vi "Targeting VI.vi"(0 "Upper Limit":T1, 4 "Lower Limit":T1, 6 "RobotDriveDevRef":T7={"DevStatus"={"status"=FALSE, "code"=0, "source"=""}, "Motors[]"=[], "Square Inputs"=FALSE, "Max Output"=1.0, "Isochronous"=FALSE}, 7 "Elevator Control":T8={"DeviceStatus"={"status"=FALSE, "code"=0, "source"=""}, "Type"=enum."PWM", "PWM"={"Digital Module"=enum."Digital Module 1", "PWM Channel"=enum."Invalid", "DeadBand"={"Name"="", "maxPositivePwm"=0, "minPositivePwm"=0, "centerPwm"=0, "maxNegativePwm"=0, "minNegativePwm"=0, "angularRange"=0}}, "CAN"={"Device Number"=0, "Control Mode"=enum."Percent VBus", "Semaphore"=refnum, "Max Vout"=12.0}, "Invert"=FALSE, "TransformRef"=refnum, "InvTransformRef"=refnum}, 8 "DO 14 LED":T14, 9 "Shoot":T4={"DevStatus"={"status"=FALSE, "code"=0, "source"=""}, "Solenoid Module"=enum."Solenoid Module 1", "Forward Solenoid Channel"=enum."Invalid", "Reverse Solenoid Channel"=enum."Invalid"}, 10 "slow turn":dbl=0.5, 11 "Aim Button":bool) -> ()   [LabVIEW 2012]
uses:
  <vilib>/Rock Robotics/WPI/DigitalOutput/WPI_DigitalOutputDevRef.ctl
  <vilib>/Rock Robotics/SystemInterfaces/Typedef/FPGA_TypedefDigitalModule.ctl
  <vilib>/Rock Robotics/SystemInterfaces/DIO/FPGA_DIOChannel.ctl
  <vilib>/Rock Robotics/WPI/MotorControl/WPI_MotorControlDeviceRef.ctl
  <vilib>/Rock Robotics/SystemInterfaces/DIO/FPGA_DIOPWMChannel.ctl
  <vilib>/Rock Robotics/WPI/PWM/WPI_PWMDeadband.ctl
  <vilib>/Rock Robotics/WPI/CAN/Jaguar/SubVIs/WPI_CANJaguar_ControlMode.ctl
  <vilib>/Rock Robotics/WPI/PWM/WPI_PWMTransform_ConPane.ctl
  <vilib>/Rock Robotics/WPI/RobotDrive/WPI_RobotDriveDevRef.ctl
  <vilib>/Rock Robotics/WPI/Solenoid/WPI_SolenoidDevRef.ctl
  <vilib>/Rock Robotics/SystemInterfaces/Typedef/FPGA_TypedefSolenoidModule.ctl
  <vilib>/Rock Robotics/WPI/Solenoid/WPI_SolenoidChannel.ctl
  <vilib>/Rock Robotics/WPI/DigitalInput/WPI_DigitalInputDevRef.ctl
  <vilib>/Rock Robotics/WPI/Solenoid/WPI_SolenoidValue.ctl
  Robot Global Data.vi
  <vilib>/Rock Robotics/WPI/Solenoid/WPI_SolenoidSetEnum.vi
panel:
  in  "lower limit Y":dbl=0.48
  in  "upper limit Y":dbl=0.5
  in  "upper limit X":dbl=0.1
  in  "lower limit X":dbl=-0.1
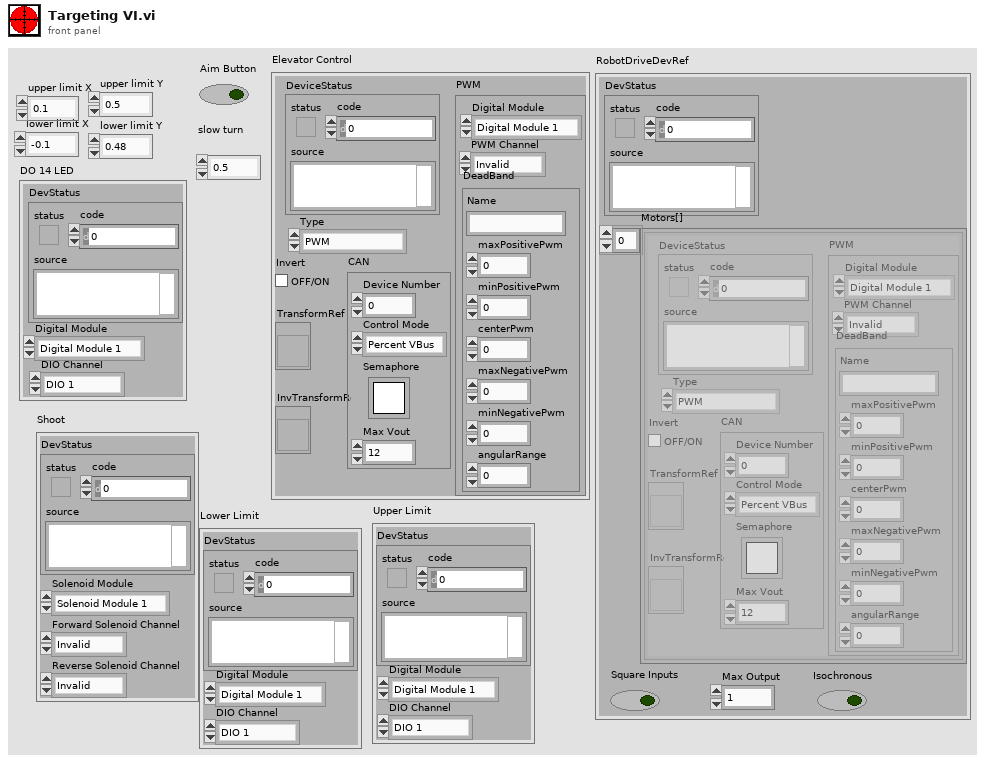
[diagram p1: front panel]
types:
  T1 = typedef "WPI_DigitalInputDevRef.ctl" = cluster{"DevStatus":errorcluster, "DIO Channel":T2, "Digital Module":T3}
  T2 = typedef "FPGA_DIOChannel.ctl" = enum8{"DIO 1", "DIO 2", "DIO 3", "DIO 4", "DIO 5", "DIO 6", "DIO 7", "DIO 8", "DIO 9", "DIO 10", "DIO 11", "DIO 12", "DIO 13", "DIO 14", "Invalid"}
  T3 = typedef "FPGA_TypedefDigitalModule.ctl" = enum16{"Digital Module 1", "Digital Module 2"}
  T4 = typedef "WPI_SolenoidDevRef.ctl" = cluster{"DevStatus":errorcluster, "Solenoid Module":T5, "Forward Solenoid Channel":T6, "Reverse Solenoid Channel":T6}
  T5 = typedef "FPGA_TypedefSolenoidModule.ctl" = enum16{"Solenoid Module 1", "Solenoid Module 2"}
  T6 = typedef "WPI_SolenoidChannel.ctl" = enum8{"Solenoid 1", "Solenoid 2", "Solenoid 3", "Solenoid 4", "Solenoid 5", "Solenoid 6", "Solenoid 7", "Solenoid 8", "Invalid"}
  T7 = typedef "WPI_RobotDriveDevRef.ctl" = cluster{"DevStatus":errorcluster, "Motors[]":T8[], "Square Inputs":bool, "Max Output":dbl, "Isochronous":bool}
  T8 = typedef "WPI_MotorControlDeviceRef.ctl" = cluster{"DeviceStatus":errorcluster, "Type":enum16{"PWM", "CAN"}, "PWM":cluster{"Digital Module":T3, "PWM Channel":T9, "DeadBand":T10}, "CAN":cluster{"Device Number":u8, "Control Mode":T11, "Semaphore":T12, "Max Vout":dbl}, "Invert":bool, "TransformRef":T13, "InvTransformRef":T13}
  T9 = typedef "FPGA_DIOPWMChannel.ctl" = enum8{"PWM 1", "PWM 2", "PWM 3", "PWM 4", "PWM 5", "PWM 6", "PWM 7", "PWM 8", "PWM 9", "PWM 10", "Invalid"}
  T10 = typedef "WPI_PWMDeadband.ctl" = cluster{"Name":string, "maxPositivePwm":i32, "minPositivePwm":i32, "centerPwm":i32, "maxNegativePwm":i32, "minNegativePwm":i32, "angularRange":u16}
  T11 = typedef "WPI_CANJaguar_ControlMode.ctl" = enum8{"Percent VBus", "Current", "Speed", "Position", "Voltage"}
  T12 = typedef "Semaphore RefNum" = refnum<k1>
  T13 = typedef "WPI_PWMTransform_ConPane.ctl" = refnum<vi>
  T14 = typedef "WPI_DigitalOutputDevRef.ctl" = cluster{"Digital Module":T3, "DIO Channel":T2, "DevStatus":errorcluster}
  T15 = cluster{"Center Position":cluster{"X":dbl, "Y":dbl}, "Distance (ft)":dbl, "Center":bool}[]
  T16 = cluster{"Center Position":cluster{"X":dbl, "Y":dbl}, "Distance (ft)":dbl, "Center":bool}
  T17 = typedef "WPI_SolenoidValue.ctl" = enum16{"Off", "On", "Forward", "Reverse"}
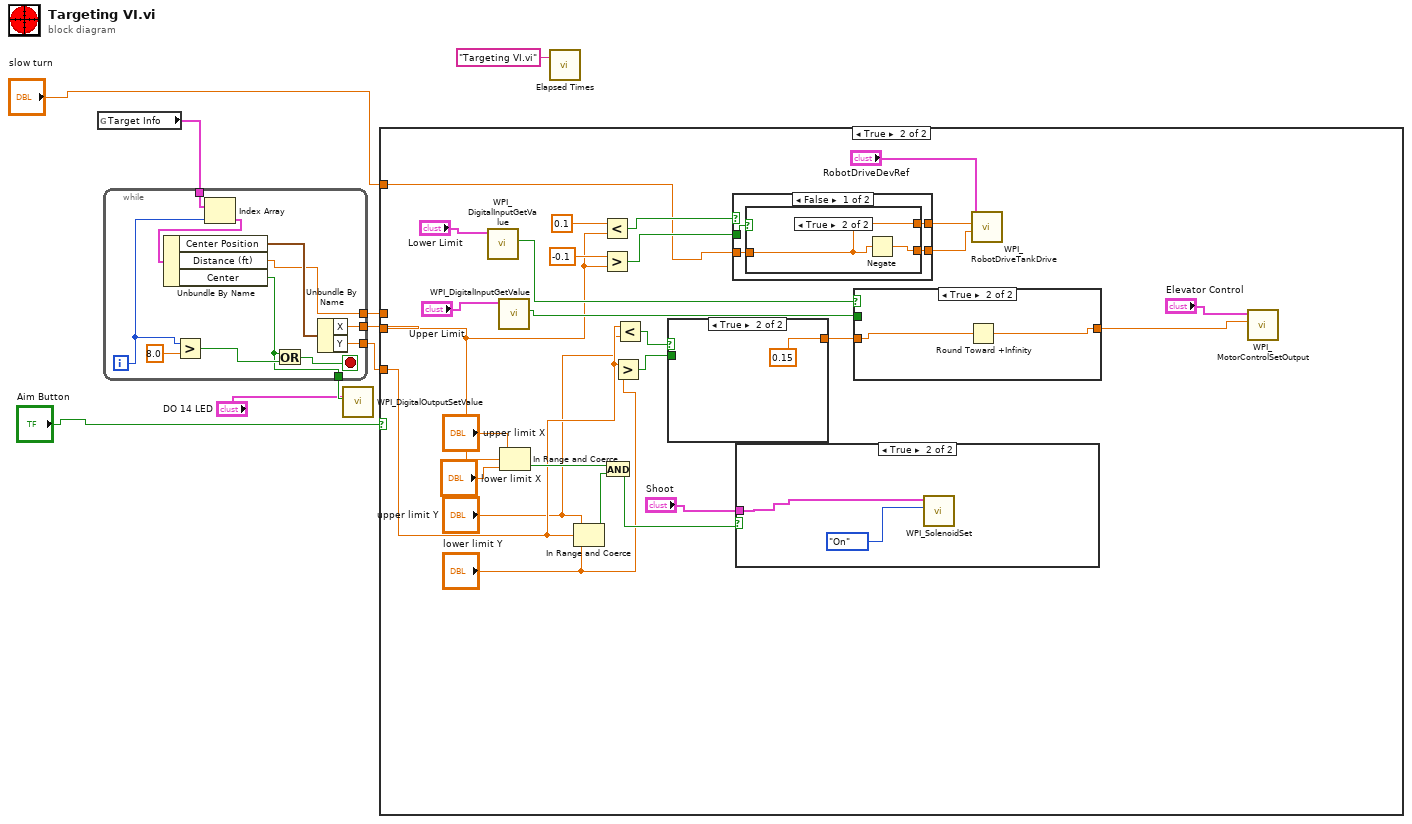
[diagram p0: block diagram]
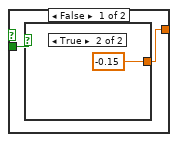
[diagram p3: hidden frame]
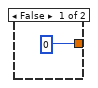
[diagram p4: hidden frame]
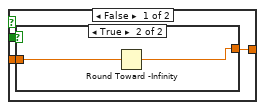
[diagram p5: hidden frame]
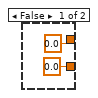
[diagram p7: hidden frame]
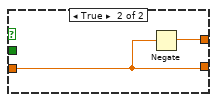
[diagram p8: hidden frame]
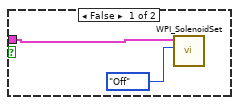
[diagram p9: hidden frame]
diagram:
  n1 = global read "Robot Global Data.vi" "Target Info"() -> (w9:T15)
  n2 = while {
    tunnel: [w19] -> w7
    tunnel: [w18] -> w6
    tunnel: w9 -> [w17]
    tunnel: [w11] -> w8
    tunnel: [w10] -> w1
    i -> [w12]
    stop <- w15 stop-if-true
    n3 = Greater?(x=w12, y=8.0) -> (0:w14:bool)
    n4 = Index Array(array=w17, index=w12) -> (element=w16:T16)
    n5 = Unbundle By Name(w16) -> ("Center Position"=w20:cluster{"X":dbl, "Y":dbl}, "Distance (ft)"=w10:dbl, "Center"=w11:bool)
    n6 = Or(x=w11, y=w14) -> (x .or. y?=w15:bool)
    n7 = Unbundle By Name(w20) -> ("X"=w18:dbl, "Y"=w19:dbl)
  }
  n8 = call <vilib>:"WPI_DigitalOutputSetValue.vi"("Value"=w8, "DigitalOutputDevRef"="DO 14 LED") -> ()  [unwired: 8 in, 2 out]
  n9 = case shown="True" "Aim Button" {
    tunnel: w7 -> [_ w23]
    tunnel: w6 -> [_ w37]
    tunnel: "slow turn" -> [_ w40]
    tunnel: w1 -> [_ _]
    frame False {
    }
    frame True {
      n10 = call <vilib>:"WPI_DigitalInputGetValue.vi"("DigitalInputDevRef"="Lower Limit") -> ("Value"=w39:bool)  [unwired: 8 in, 2 out]
      n11 = call <vilib>:"WPI_DigitalInputGetValue.vi"("DigitalInputDevRef"="Upper Limit") -> ("Value"=w38:bool)  [unwired: 8 in, 2 out]
      n12 = In Range and Coerce(upper limit="upper limit X", x=w37, lower limit="lower limit X") -> (In Range?=w35:bool)  [unwired: 1 out]
      n13 = In Range and Coerce(upper limit="upper limit Y", x=w23, lower limit="lower limit Y") -> (In Range?=w36:bool)  [unwired: 1 out]
      n14 = Less?(x=0.1, y=w37) -> (x < y?=w42:bool)
      n15 = Greater?(x=-0.1, y=w37) -> (0:w41:bool)
      n16 = And(x=w35, y=w36) -> (x .and. y?=w43:bool)
      n17 = Greater?(x=w23, y="lower limit Y") -> (0:w25:bool)
      n18 = Less?(x=w23, y="upper limit Y") -> (x < y?=w26:bool)
      n19 = case shown="True" w26 {
        tunnel: w25 -> [w49 _]
        tunnel: [w48 0.15] -> w24
        frame False {
          n20 = case shown="True" w49 {
            tunnel: [0 -0.15] -> w48
            frame False {
            }
            frame True {
            }
          }
        }
        frame True {
        }
      }
      n21 = case shown="False" w42 {
        tunnel: [w64 w70] -> w45
        tunnel: [w62 w69] -> w44
        tunnel: w40 -> [w63 w69]
        tunnel: w41 -> [w61 _]
        frame False {
          n22 = case shown="True" w61 {
            tunnel: [0.0 w67] -> w64
            tunnel: w63 -> [_ w67]
            tunnel: [0.0 w68] -> w62
            frame False {
            }
            frame True {
              n23 = Negate(x=w67) -> (-x=w68:dbl)
            }
          }
        }
        frame True {
          n24 = Negate(x=w69) -> (-x=w70:dbl)
        }
      }
      n25 = case shown="True" w43 {
        tunnel: "Shoot" -> [w71 w74]
        frame False {
          n26 = call-poly <vilib>:"WPI_SolenoidSet.vi"("Value"=WPI_SolenoidValue."Off", "SolenoidDevRef"=w71) -> ()  [unwired: 8 in, 2 out]
        }
        frame True {
          n27 = call-poly <vilib>:"WPI_SolenoidSet.vi"("Value"=WPI_SolenoidValue."On", "SolenoidDevRef"=w74) -> ()  [unwired: 8 in, 2 out]
        }
      }
      n28 = case shown="True" w39 {
        tunnel: w38 -> [w54 _]
        tunnel: [w55 w60] -> w32
        tunnel: w24 -> [w53 w59]
        frame False {
          n29 = case shown="True" w54 {
            tunnel: [w56 w58] -> w55
            tunnel: w53 -> [w56 w57]
            frame False {
            }
            frame True {
              n30 = Round Toward -Infinity(1:w57) -> (0:w58:dbl)
            }
          }
        }
        frame True {
          n31 = Round Toward +Infinity(x=w59) -> (ceil(x): smallest int >= x=w60:dbl)
        }
      }
      n32 = call <vilib>:"WPI_RobotDriveTankDrive.vi"("Right axis value"=w44, "Left axis value"=w45, "RobotDriveDevRef"="RobotDriveDevRef") -> ()  [unwired: 6 in, 3 out]
      n33 = call <vilib>:"WPI_MotorControlSetOutput.vi"("Output"=w32, "MotorControlDevRef"="Elevator Control") -> ()  [unwired: 7 in, 3 out]
    }
  }
  n34 = call "Elapsed Times.vi"("Call Name"="Targeting VI.vi") -> ()  [unwired: 2 in, 1 out]
